vi "AddNetworkCredentials.vi"(6 "Domain":string, 8 "error in (no error)":errorcluster, 9 "password":string, 10 "userName":string, 11 "WebProxy_NET in":refnum<class "WebProxy_NET.lvclass">) -> (0 "error out":errorcluster, 3 "WebProxy_NET out":refnum<class "WebProxy_NET.lvclass">)   [LabVIEW 2018, in "LabVIEWHTTPClient_NET.lvlib" / "WebProxy_NET.lvclass"]
uses:
  WebProxy_NET.lvclass
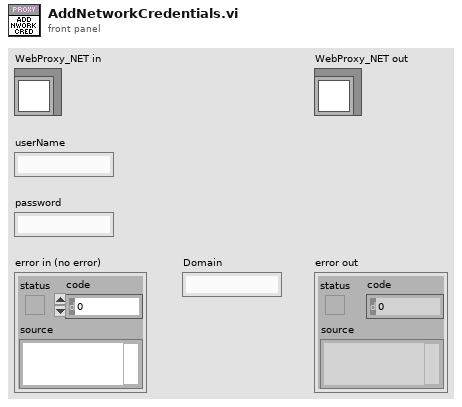
[diagram p1: front panel]
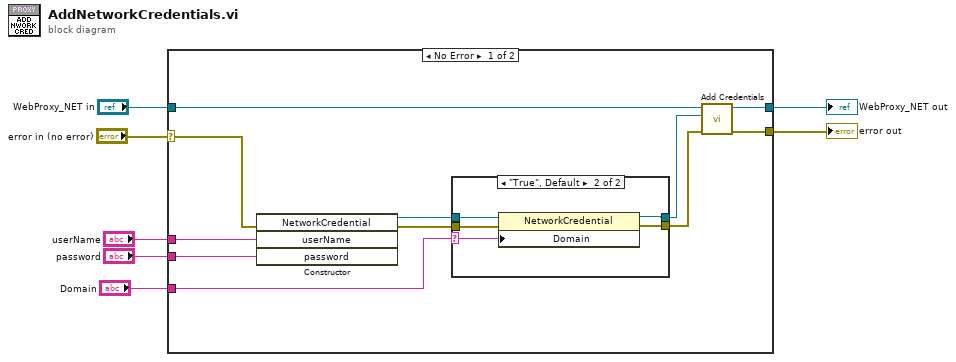
[diagram p0: block diagram]
diagram:
  n1 = case shown="No Error" "error in (no error)" {
    selector: "error in (no error)" -> [w9 w27]
    tunnel: "WebProxy_NET in" -> [w18 w26]
    tunnel: "userName" -> [w16 _]
    tunnel: "password" -> [w15 _]
    tunnel: "Domain" -> [w14 _]
    tunnel: [w12 w26] -> w3
    tunnel: [w8 w27] -> w1
    frame No Error {
      n2 = constructor class="NetworkCredential"(error in=w9, "userName"=w16, "password"=w15) -> (reference out=w17:refnum<k24>, error out=w13:errorcluster)  [unwired: 2 in, 3 out]
      n3 = case shown="\"True\", Default" w14 {
        selector: w14 -> [_ w24]
        tunnel: w17 -> [w20 w25]
        tunnel: [w20 w23] -> w11
        tunnel: w13 -> [w19 w22]
        tunnel: [w19 w21] -> w10
        frame "" {
        }
        frame "True", Default {
          n4 = property class="NetworkCredential"(reference=w25, error in=w22, "Domain"=w24) -> (reference out=w23:refnum<k24>, error out=w21:errorcluster)
        }
      }
      n5 = call "Add Credentials.vi"("error in (no error)"=w10, "Credentials"=w11, "WebProxy_NET in"=w18) -> ("error out"=w8:errorcluster, "WebProxy_NET out"=w12:refnum<class "WebProxy_NET.lvclass">)  [unwired: 7 in]
    }
    frame Error {
    }
  }
  "error out" <- w1
  "WebProxy_NET out" <- w3
